vi "Lab Panel V4.91.vi"() -> ()   [LabVIEW 2013] (continued)
                }
              }
              frame #3 {
                # "LAB02-2"
                n2516 = case shown="True" w4752 {
                  tunnel: w4754 -> [_ w4767]
                  tunnel: w4751 -> [_ w4764]
                  tunnel: w4753 -> [_ w4763]
                  frame False {
                  }
                  frame True {
                    n2517 = local read "TEMP START LAB02-2"() -> (w4769:cluster{"TL":dbl, "TN":dbl})
                    n2518 = local read "FAIL LAB02-2"() -> (w4760:cluster{"LO":dbl, "HI":dbl})
                    n2519 = local read "TDMS LAB02-2"() -> (w4768:refnum<k34>)
                    n2520 = local read "SET LAB02-2"() -> (w4765:T5)
                    n2521 = local read "DISP LAB02-2"() -> (w4766:T4)
                    n2522 = local read "SIG LAB02-2"() -> (w4770:T2)
                    n2523 = local read "RESULT LAB02-2"() -> (w4757:bool)
                    n2524 = Bundle("FAIL LAB02-2"=w4760, "SIG LAB02-2"=w4770, "TEMP START LAB02-2"=w4769, "DISP LAB02-2"=w4766, "SET LAB02-2"=w4765, "TDMS LAB02-2"=w4768) -> (w4755:T35)  [unwired: 1 in]
                    n2525 = call "sub vi - cycle&temp fail v7.vi"("Amps Lo?"=w4767, "Input Cluster"=w4755, "SELECT"=w4764, "Amps Hi?"=w4763, "Result In"=w4757) -> ("(FAIL) out"=w4759:cluster{"FAIL LO":dbl, "FAIL HI":dbl}, "(DISP) out"=w4762:T4, "T-RISE"=w4756:cluster{"T-RISE (L)":dbl, "T-RISE (N)":dbl}, "Result Out"=w4758:bool, "file error"=w4761:errorcluster)  [unwired: 10 in]
                    n2526 = local write "TEMP RISE LAB02-2"(w4756) -> ()
                    n2527 = local write "FAIL LAB02-2"(w4759) -> ()
                    n2528 = local write "DISP LAB02-2"(w4762) -> ()
                    n2529 = local write "RESULT LAB02-2"(w4758) -> ()
                    n2530 = local write "data file error"(w4761) -> ()
                  }
                }
              }
              frame #4 {
                # "LAB03-1"
                n2531 = case shown="True" w4772 {
                  tunnel: w4774 -> [_ w4787]
                  tunnel: w4771 -> [_ w4784]
                  tunnel: w4773 -> [_ w4783]
                  frame False {
                  }
                  frame True {
                    n2532 = local read "TEMP START LAB03-1"() -> (w4789:cluster{"TL":dbl, "TN":dbl})
                    n2533 = local read "FAIL LAB03-1"() -> (w4780:cluster{"LO":dbl, "HI":dbl})
                    n2534 = local read "TDMS LAB03-1"() -> (w4788:refnum<k34>)
                    n2535 = local read "SET LAB03-1"() -> (w4785:T5)
                    n2536 = local read "DISP LAB03-1"() -> (w4786:T4)
                    n2537 = local read "SIG LAB03-1"() -> (w4790:T2)
                    n2538 = local read "RESULT LAB03-1"() -> (w4777:bool)
                    n2539 = Bundle("FAIL LAB03-1"=w4780, "SIG LAB03-1"=w4790, "TEMP START LAB03-1"=w4789, "DISP LAB03-1"=w4786, "SET LAB03-1"=w4785, "TDMS LAB03-1"=w4788) -> (w4775:T36)  [unwired: 1 in]
                    n2540 = call "sub vi - cycle&temp fail v7.vi"("Amps Lo?"=w4787, "Input Cluster"=w4775, "SELECT"=w4784, "Amps Hi?"=w4783, "Result In"=w4777) -> ("(FAIL) out"=w4779:cluster{"FAIL LO":dbl, "FAIL HI":dbl}, "(DISP) out"=w4782:T4, "T-RISE"=w4776:cluster{"T-RISE (L)":dbl, "T-RISE (N)":dbl}, "Result Out"=w4778:bool, "file error"=w4781:errorcluster)  [unwired: 10 in]
                    n2541 = local write "TEMP RISE LAB03-1"(w4776) -> ()
                    n2542 = local write "FAIL LAB03-1"(w4779) -> ()
                    n2543 = local write "DISP LAB03-1"(w4782) -> ()
                    n2544 = local write "RESULT LAB03-1"(w4778) -> ()
                    n2545 = local write "data file error"(w4781) -> ()
                  }
                }
              }
              frame #5 {
                # "LAB03-2"
                n2546 = case shown="True" w4792 {
                  tunnel: w4794 -> [_ w4807]
                  tunnel: w4791 -> [_ w4804]
                  tunnel: w4793 -> [_ w4803]
                  frame False {
                  }
                  frame True {
                    n2547 = local read "TEMP START LAB03-2"() -> (w4809:cluster{"TL":dbl, "TN":dbl})
                    n2548 = local read "FAIL LAB03-2"() -> (w4800:cluster{"LO":dbl, "HI":dbl})
                    n2549 = local read "TDMS LAB03-2"() -> (w4808:refnum<k34>)
                    n2550 = local read "SET LAB03-2"() -> (w4805:T5)
                    n2551 = local read "DISP LAB03-2"() -> (w4806:T4)
                    n2552 = local read "RESULT LAB03-2"() -> (w4797:bool)
                    n2553 = local read "SIG LAB03-2"() -> (w4810:T2)
                    n2554 = Bundle("FAIL LAB03-2"=w4800, "SIG LAB03-2"=w4810, "TEMP START LAB03-2"=w4809, "DISP LAB03-2"=w4806, "SET LAB03-2"=w4805, "TDMS LAB03-2"=w4808) -> (w4795:T37)  [unwired: 1 in]
                    n2555 = call "sub vi - cycle&temp fail v7.vi"("Amps Lo?"=w4807, "Input Cluster"=w4795, "SELECT"=w4804, "Amps Hi?"=w4803, "Result In"=w4797) -> ("(FAIL) out"=w4799:cluster{"FAIL LO":dbl, "FAIL HI":dbl}, "(DISP) out"=w4802:T4, "T-RISE"=w4796:cluster{"T-RISE (L)":dbl, "T-RISE (N)":dbl}, "Result Out"=w4798:bool, "file error"=w4801:errorcluster)  [unwired: 10 in]
                    n2556 = local write "FAIL LAB03-2"(w4799) -> ()
                    n2557 = local write "TEMP RISE LAB03-2"(w4796) -> ()
                    n2558 = local write "DISP LAB03-2"(w4802) -> ()
                    n2559 = local write "RESULT LAB03-2"(w4798) -> ()
                    n2560 = local write "data file error"(w4801) -> ()
                  }
                }
              }
              frame #6 {
                # "LAB04-1"
                n2561 = case shown="True" w4812 {
                  tunnel: w4814 -> [_ w4827]
                  tunnel: w4811 -> [_ w4824]
                  tunnel: w4813 -> [_ w4823]
                  frame False {
                  }
                  frame True {
                    n2562 = local read "TEMP START LAB04-1"() -> (w4829:cluster{"TL":dbl, "TN":dbl})
                    n2563 = local read "FAIL LAB04-1"() -> (w4820:cluster{"LO":dbl, "HI":dbl})
                    n2564 = local read "TDMS LAB04-1"() -> (w4828:refnum<k34>)
                    n2565 = local read "SET LAB04-1"() -> (w4825:T5)
                    n2566 = local read "DISP LAB04-1"() -> (w4826:T4)
                    n2567 = local read "SIG LAB04-1"() -> (w4830:T2)
                    n2568 = local read "RESULT LAB04-1"() -> (w4817:bool)
                    n2569 = Bundle("FAIL LAB04-1"=w4820, "SIG LAB04-1"=w4830, "TEMP START LAB04-1"=w4829, "DISP LAB04-1"=w4826, "SET LAB04-1"=w4825, "TDMS LAB04-1"=w4828) -> (w4815:T38)  [unwired: 1 in]
                    n2570 = call "sub vi - cycle&temp fail v7.vi"("Amps Lo?"=w4827, "Input Cluster"=w4815, "SELECT"=w4824, "Amps Hi?"=w4823, "Result In"=w4817) -> ("(FAIL) out"=w4819:cluster{"FAIL LO":dbl, "FAIL HI":dbl}, "(DISP) out"=w4822:T4, "T-RISE"=w4816:cluster{"T-RISE (L)":dbl, "T-RISE (N)":dbl}, "Result Out"=w4818:bool, "file error"=w4821:errorcluster)  [unwired: 10 in]
                    n2571 = local write "TEMP RISE LAB04-1"(w4816) -> ()
                    n2572 = local write "FAIL LAB04-1"(w4819) -> ()
                    n2573 = local write "DISP LAB04-1"(w4822) -> ()
                    n2574 = local write "RESULT LAB04-1"(w4818) -> ()
                    n2575 = local write "data file error"(w4821) -> ()
                  }
                }
              }
              frame #7 {
                # "LAB04-2"
                n2576 = case shown="True" w4832 {
                  tunnel: w4834 -> [_ w4847]
                  tunnel: w4831 -> [_ w4844]
                  tunnel: w4833 -> [_ w4843]
                  frame False {
                  }
                  frame True {
                    n2577 = local read "TEMP START LAB04-2"() -> (w4849:cluster{"TL":dbl, "TN":dbl})
                    n2578 = local read "FAIL LAB04-2"() -> (w4840:cluster{"LO":dbl, "HI":dbl})
                    n2579 = local read "TDMS LAB04-2"() -> (w4848:refnum<k34>)
                    n2580 = local read "SET LAB04-2"() -> (w4845:T5)
                    n2581 = local read "DISP LAB04-2"() -> (w4846:T4)
                    n2582 = local read "SIG LAB04-2"() -> (w4850:T2)
                    n2583 = local read "RESULT LAB04-2"() -> (w4837:bool)
                    n2584 = Bundle("FAIL LAB04-2"=w4840, "SIG LAB04-2"=w4850, "TEMP START LAB04-2"=w4849, "DISP LAB04-2"=w4846, "SET LAB04-2"=w4845, "TDMS LAB04-2"=w4848) -> (w4835:T39)  [unwired: 1 in]
                    n2585 = call "sub vi - cycle&temp fail v7.vi"("Amps Lo?"=w4847, "Input Cluster"=w4835, "SELECT"=w4844, "Amps Hi?"=w4843, "Result In"=w4837) -> ("(FAIL) out"=w4839:cluster{"FAIL LO":dbl, "FAIL HI":dbl}, "(DISP) out"=w4842:T4, "T-RISE"=w4836:cluster{"T-RISE (L)":dbl, "T-RISE (N)":dbl}, "Result Out"=w4838:bool, "file error"=w4841:errorcluster)  [unwired: 10 in]
                    n2586 = local write "TEMP RISE LAB04-2"(w4836) -> ()
                    n2587 = local write "FAIL LAB04-2"(w4839) -> ()
                    n2588 = local write "DISP LAB04-2"(w4842) -> ()
                    n2589 = local write "RESULT LAB04-2"(w4838) -> ()
                    n2590 = local write "data file error"(w4841) -> ()
                  }
                }
              }
              frame #8 {
                # "LAB05-1"
                n2591 = case shown="True" w4852 {
                  tunnel: w4854 -> [_ w4867]
                  tunnel: w4851 -> [_ w4864]
                  tunnel: w4853 -> [_ w4863]
                  frame False {
                  }
                  frame True {
                    n2592 = local read "TEMP START LAB05-1"() -> (w4869:cluster{"TL":dbl, "TN":dbl})
                    n2593 = local read "FAIL LAB05-1"() -> (w4860:cluster{"LO":dbl, "HI":dbl})
                    n2594 = local read "TDMS LAB05-1"() -> (w4868:refnum<k34>)
                    n2595 = local read "SET LAB05-1"() -> (w4865:T5)
                    n2596 = local read "DISP LAB05-1"() -> (w4866:T4)
                    n2597 = local read "SIG LAB05-1"() -> (w4870:T2)
                    n2598 = local read "RESULT LAB05-1"() -> (w4857:bool)
                    n2599 = Bundle("FAIL LAB05-1"=w4860, "SIG LAB05-1"=w4870, "TEMP START LAB05-1"=w4869, "DISP LAB05-1"=w4866, "SET LAB05-1"=w4865, "TDMS LAB05-1"=w4868) -> (w4855:T40)  [unwired: 1 in]
                    n2600 = call "sub vi - cycle&temp fail v7.vi"("Amps Lo?"=w4867, "Input Cluster"=w4855, "SELECT"=w4864, "Amps Hi?"=w4863, "Result In"=w4857) -> ("(FAIL) out"=w4859:cluster{"FAIL LO":dbl, "FAIL HI":dbl}, "(DISP) out"=w4862:T4, "T-RISE"=w4856:cluster{"T-RISE (L)":dbl, "T-RISE (N)":dbl}, "Result Out"=w4858:bool, "file error"=w4861:errorcluster)  [unwired: 10 in]
                    n2601 = local write "TEMP RISE LAB05-1"(w4856) -> ()
                    n2602 = local write "FAIL LAB05-1"(w4859) -> ()
                    n2603 = local write "DISP LAB05-1"(w4862) -> ()
                    n2604 = local write "RESULT LAB05-1"(w4858) -> ()
                    n2605 = local write "data file error"(w4861) -> ()
                  }
                }
              }
              frame #9 {
                # "LAB05-2"
                n2606 = case shown="True" w4872 {
                  tunnel: w4874 -> [_ w4887]
                  tunnel: w4871 -> [_ w4884]
                  tunnel: w4873 -> [_ w4883]
                  frame False {
                  }
                  frame True {
                    n2607 = local read "TEMP START LAB05-2"() -> (w4889:cluster{"TL":dbl, "TN":dbl})
                    n2608 = local read "FAIL LAB05-2"() -> (w4880:cluster{"LO":dbl, "HI":dbl})
                    n2609 = local read "TDMS LAB05-2"() -> (w4888:refnum<k34>)
                    n2610 = local read "SET LAB05-2"() -> (w4885:T5)
                    n2611 = local read "DISP LAB05-2"() -> (w4886:T4)
                    n2612 = local read "SIG LAB05-2"() -> (w4890:T2)
                    n2613 = local read "RESULT LAB05-2"() -> (w4877:bool)
                    n2614 = Bundle("FAIL LAB05-2"=w4880, "SIG LAB05-2"=w4890, "TEMP START LAB05-2"=w4889, "DISP LAB05-2"=w4886, "SET LAB05-2"=w4885, "TDMS LAB05-2"=w4888) -> (w4875:T41)  [unwired: 1 in]
                    n2615 = call "sub vi - cycle&temp fail v7.vi"("Amps Lo?"=w4887, "Input Cluster"=w4875, "SELECT"=w4884, "Amps Hi?"=w4883, "Result In"=w4877) -> ("(FAIL) out"=w4879:cluster{"FAIL LO":dbl, "FAIL HI":dbl}, "(DISP) out"=w4882:T4, "T-RISE"=w4876:cluster{"T-RISE (L)":dbl, "T-RISE (N)":dbl}, "Result Out"=w4878:bool, "file error"=w4881:errorcluster)  [unwired: 10 in]
                    n2616 = local write "TEMP RISE LAB05-2"(w4876) -> ()
                    n2617 = local write "FAIL LAB05-2"(w4879) -> ()
                    n2618 = local write "DISP LAB05-2"(w4882) -> ()
                    n2619 = local write "RESULT LAB05-2"(w4878) -> ()
                    n2620 = local write "data file error"(w4881) -> ()
                  }
                }
              }
            }
          }
          frame #15 {
            # "run calibration routine"
            n2621 = local read "SET (cal)"() -> (w4891:bool)
            n2622 = case shown="True" w4891 {
              frame False {
              }
              frame True {
                n2623 = stacked-sequence {
                  seq-local: [w4892 _ _] -> [_ w4894 _]
                  frame #0 {
                    n2624 = call "CALIBRATION PASSWORD"() -> ("PASSWORD"=w4892:string)  [unwired: 17 in, 2 out]
                  }
                  frame #1 {
                    n2625 = Equal?(x=w4894, y="7777") -> (x = y?=w4893:bool)
                    n2626 = case shown="True" w4893 {
                      frame False {
                      }
                      frame True {
                        n2627 = stacked-sequence {
                          frame #0 {
                            n2628 = local read "Temp Test Cal"() -> (w4896:dbl)
                            n2629 = call "sub vi - calibration v1.vi"("Temp Test Cal"=w4896) -> ()  [unwired: 11 in]
                          }
                          frame #1 {
                            n2630 = call "sub vi - get calibration values v1.vi"() -> ("TEMP REF CAL"=w4897:dbl, "LAB01 (CAL)"=w4902:T14, "LAB02 (CAL)"=w4901:T15, "LAB03 (CAL)"=w4900:T14, "LAB04 (CAL)"=w4899:T14, "calibration file error out"=w4903:errorcluster, "LAB05 (CAL)"=w4898:T14)  [unwired: 9 in]
                            n2631 = local write "TEMP REF cal"(w4897) -> ()
                            n2632 = local write "cal file error out"(w4903) -> ()
                            n2633 = local write "CAL LAB04"(w4899) -> ()
                            n2634 = local write "CAL LAB05"(w4898) -> ()
                            n2635 = local write "CAL LAB01"(w4902) -> ()
                            n2636 = local write "CAL LAB02"(w4901) -> ()
                            n2637 = local write "CAL LAB03"(w4900) -> ()
                          }
                        }
                      }
                    }
                  }
                  frame #2 {
                    n2638 = local write "SET (cal)"(FALSE) -> ()
                  }
                }
              }
            }
          }
          frame #16 {
            # "save certain settings to file"
            n2639 = String To Path(string="c:\\crabtree\\Set Up\\") -> (path=w4906:path)
            n2640 = Build Path(base path=w4906, name or relative path="settings.bin") -> (appended path=w4908:path)
            n2641 = Build Path(base path=w4906, name or relative path="mail.bin") -> (appended path=w4905:path)
            n2642 = Create Folder(path (use dialog)=w4906) -> (error out=w4911:errorcluster)  [unwired: 2 in, 2 out]
            n2643 = call <vilib>:"Clear Errors.vi"("error in (no error)"=w4911) -> ()  [unwired: 6 in, 1 out]
            n2644 = stacked-sequence {
              seq-local: [w4923 _] -> [_ w4936]
              tunnel: w4908 -> [_ w4937]
              tunnel: w4905 -> [_ w4935]
              frame #0 {
                n2645 = local read "C drive data root dir"() -> (w4922:path)
                n2646 = local read "Select COM port"() -> (w4919:refnum<visa-resource-name>)
                n2647 = local read "Network Directory"() -> (w4928:path)
                n2648 = local read "SET LAB05-2"() -> (w4927:T5)
                n2649 = local read "SET LAB05-1"() -> (w4926:T5)
                n2650 = local read "SET LAB04-2"() -> (w4925:T5)
                n2651 = local read "SET LAB03-2"() -> (w4929:T5)
                n2652 = local read "SET LAB04-1"() -> (w4924:T5)
                n2653 = local read "SET LAB03-1"() -> (w4930:T5)
                n2654 = local read "SET LAB02-2"() -> (w4931:T5)
                n2655 = local read "SET LAB02-1"() -> (w4932:T5)
                n2656 = local read "Temp Delay Lps"() -> (w4918:dbl)
                n2657 = local read "Amps Fail level"() -> (w4914:dbl)
                n2658 = local read "SET LAB01-2"() -> (w4933:T5)
                n2659 = local read "Temp Test Cal"() -> (w4915:dbl)
                n2660 = local read "SET LAB01-1"() -> (w4934:T5)
                n2661 = local read "Mail Test File To:"() -> (w4913:string)
                n2662 = local read "Temp Value"() -> (w4917:dbl)
                n2663 = local read "Fail Loops"() -> (w4916:dbl)
                n2664 = local read "Mail Test Fail"() -> (w4912:bool)
                n2665 = local read "RATE (Hz)"() -> (w4921:dbl)
                n2666 = local read "SAMPLES"() -> (w4920:dbl)
                n2667 = Bundle("SET LAB01-1"=w4934, "SET LAB01-2"=w4933, "SET LAB02-1"=w4932, "SET LAB02-2"=w4931, "SET LAB03-1"=w4930, "SET LAB03-2"=w4929, "SET LAB04-1"=w4924, "SET LAB04-2"=w4925, "SET LAB05-1"=w4926, "SET LAB05-2"=w4927, "Network Directory"=w4928, "C drive data root dir"=w4922, "RATE (Hz)"=w4921, "SAMPLES"=w4920, "Select COM port"=w4919, "Temp Delay Lps"=w4918, "Temp Value"=w4917, "Fail Loops"=w4916, "Temp Test Cal"=w4915, "Amps Fail level"=w4914, "Mail Test File To:"=w4913, "Mail Test Fail"=w4912) -> (w4923:T22)  [unwired: 1 in]
              }
              frame #1 {
                n2668 = event shown="[1] \"SET LAB01-1\", \"SET LAB01-2\", \"SET LAB02-1\", \"SET LAB02-2\", \"SET LAB03-1\", \"SET LAB03-2\", \"SET LAB04-1\", \"SET LAB04-2\", \"SET LAB05-1\", \"SET LAB05-2\", \"Network Directory\", \"C drive data root dir\", \"RATE (Hz)\", \"SAMPLES\", \"Select COM port\", \"Temp Delay Lps\", \"Temp Value\", \"Fail Loops\", \"Temp Test Cal\", \"Amps Fail level\", \"Mail Test File To:\", \"Mail Test Fail\": Value Change" {
                  selector: _ -> [_ _ _]
                  dyn-events: _ -> [_ _ _]
                  timeout: 10.0 -> [_ _ _]
                  tunnel: w4937 -> [_ w4939 _]
                  tunnel: w4936 -> [_ w4940 _]
                  tunnel: w4935 -> [_ _ w4951]
                  event Timeout {
                    n2669 = event-data() -> ()  [unwired: 1 in, 3 out]
                  }
                  event "SET LAB01-1", "SET LAB01-2", "SET LAB02-1", "SET LAB02-2", "SET LAB03-1", "SET LAB03-2", "SET LAB04-1", "SET LAB04-2", "SET LAB05-1", "SET LAB05-2", "Network Directory", "C drive data root dir", "RATE (Hz)", "SAMPLES", "Select COM port", "Temp Delay Lps", "Temp Value", "Fail Loops", "Temp Test Cal", "Amps Fail level", "Mail Test File To:", "Mail Test Fail": Value Change {
                    n2670 = event-data() -> ()  [unwired: 1 in, 6 out]
                    n2671 = Open/Create/Replace File(file path (use dialog)=w4939, operation (0:open)=T21."replace or create") -> (refnum out=w4945:refnum<file>, error out=w4944:errorcluster)  [unwired: 4 in, 1 out]
                    n2672 = Write to Binary File(file (use dialog)=w4945, data=w4940, error in=w4944) -> (refnum out=w4943:refnum<file>, error out=w4942:errorcluster)  [unwired: 3 in, 1 out]
                    n2673 = Close File(refnum=w4943, error in=w4942) -> (error out=w4941:errorcluster)  [unwired: 1 out]
                    n2674 = local write "data file error"(w4941) -> ()
                  }
                  event "MAIL SETTINGS.OUT SERVER ADDRESS", "MAIL SETTINGS.FROM ACCOUNT", "MAIL SETTINGS.USER NAME", "MAIL SETTINGS.PASSWORD", "Auto Mail Send", "TO (string):": Value Change {
                    n2675 = event-data() -> ()  [unwired: 1 in, 6 out]
                    n2676 = local read "MAIL SETTINGS"() -> (w4950:T7)
                    n2677 = local read "Auto Mail Send"() -> (w4948:bool)
                    n2678 = local read "TO (string):"() -> (w4947:string)
                    n2679 = Open/Create/Replace File(file path (use dialog)=w4951, operation (0:open)=T21."replace or create") -> (refnum out=w4956:refnum<file>, error out=w4955:errorcluster)  [unwired: 4 in, 1 out]
                    n2680 = Bundle("MAIL SETTINGS"=w4950, "Auto Mail Send"=w4948, "TO (string):"=w4947) -> (w4949:T42)  [unwired: 1 in]
                    n2681 = Write to Binary File(file (use dialog)=w4956, data=w4949, error in=w4955) -> (refnum out=w4954:refnum<file>, error out=w4953:errorcluster)  [unwired: 3 in, 1 out]
                    n2682 = Close File(refnum=w4954, error in=w4953) -> (error out=w4952:errorcluster)  [unwired: 1 out]
                    n2683 = local write "data file error"(w4952) -> ()
                  }
                }
              }
            }
          }
          frame #17 {
            # "mail control"
            n2684 = local read "MAIL SETTINGS"() -> (w4973:T7)
            n2685 = local read "Auto Mail Send"() -> (w4959:bool)
            n2686 = Unbundle(w4973) -> ("OUT SERVER ADDRESS"=w4972:string, "FROM ACCOUNT"=w4971:string, "TEST MAIL"=w4970:bool)  [unwired: 4 out]
            n2687 = stacked-sequence {
              tunnel: "TO (string):" -> [_ w5012]
              tunnel: w4973 -> [w4978 w5011]
              tunnel: w4972 -> [w4977 w5010]
              tunnel: w4971 -> [w4976 w5009]
              tunnel: w4970 -> [w4975 _]
              tunnel: w4959 -> [_ w5008]
              tunnel: w4969 -> [_ w5007]
              tunnel: w4968 -> [_ w5006]
              tunnel: w4967 -> [_ w5005]
              tunnel: w4966 -> [_ w5004]
              tunnel: w4965 -> [_ w5003]
              tunnel: w4964 -> [_ w5002]
              tunnel: w4963 -> [_ w5001]
              tunnel: w4962 -> [_ w5000]
              tunnel: w4961 -> [_ w4999]
              tunnel: w4960 -> [_ w4998]
              tunnel: "TO (string):" -> [w4974 _]
              frame #0 {
                # "mail test"
                n2688 = case shown="True" w4975 {
                  tunnel: w4978 -> [_ w4982]
                  tunnel: w4974 -> [_ w4981]
                  tunnel: w4977 -> [_ w4980]
                  tunnel: w4976 -> [_ w4979]
                  frame False {
                  }
                  frame True {
                    n2689 = stacked-sequence {
                      seq-local: [_ _ w4992 _] -> [_ _ _ w4993]
                      tunnel: w4982 -> [w4985 _ _ w4997]
                      tunnel: w4981 -> [_ _ w4990 _]
                      tunnel: w4980 -> [_ _ w4988 _]
                      tunnel: w4979 -> [_ _ w4989 _]
                      frame #0 {
                        n2690 = Bundle(cluster=w4985, "TEST MAIL STATUS"="TEST START") -> (w4983:T7)  [unwired: 6 in]
                        n2691 = local write "MAIL SETTINGS"(w4983) -> ()
                      }
                      frame #1 {
                        n2692 = Wait (ms)(milliseconds to wait=500) -> ()  [unwired: 1 out]
                      }
                      frame #2 {
                        n2693 = call "sub vi - send mail v5.vi"("TO:"=w4990, "subject"="MAIL TEST FROM LAB PANEL", "from"=w4989, "out going server"=w4988, "message"="TEST MESSAGE") -> ("error out"=w4992:errorcluster)  [unwired: 10 in]
                      }
                      frame #3 {
                        n2694 = Bundle(cluster=w4997, "TEST MAIL"=FALSE, "TEST MAIL STATUS"="TEST END", "mail error"=w4993) -> (w4995:T7)  [unwired: 4 in]
                        n2695 = local write "MAIL SETTINGS"(w4995) -> ()
                      }
                    }
                  }
                }
              }
              frame #1 {
                # "mail report"
                n2696 = stacked-sequence {
                  seq-local: [_ w5055 _ _] -> [_ _ _ w5245]
                  seq-local: [_ _ w5158 _] -> [_ _ _ w5235]
                  seq-local: [w5022 _ _ _] -> [_ w5072 _ _]
                  seq-local: [w5021 _ _ _] -> [_ w5071 _ _]
                  seq-local: [w5019 _ _ _] -> [_ w5069 _ _]
                  seq-local: [w5020 _ _ _] -> [_ w5070 _ _]
                  seq-local: [w5018 _ _ _] -> [_ w5068 _ _]
                  seq-local: [w5017 _ _ _] -> [_ w5063 _ _]
                  seq-local: [w5016 _ _ _] -> [_ w5064 _ _]
                  seq-local: [w5015 _ _ _] -> [_ w5065 _ _]
                  seq-local: [w5014 _ _ _] -> [_ w5066 _ _]
                  seq-local: [w5013 _ _ _] -> [_ w5067 _ _]
                  tunnel: w5012 -> [_ _ _ w5246]
                  tunnel: w5011 -> [_ _ _ w5229]
                  tunnel: w5010 -> [_ _ _ w5243]
                  tunnel: w5009 -> [_ _ _ w5242]
                  tunnel: w5008 -> [w5053 _ _ w5237]
                  tunnel: w5007 -> [_ _ w5188 _]
                  tunnel: w5006 -> [_ _ w5185 _]
                  tunnel: w5005 -> [_ _ w5184 _]
                  tunnel: w5004 -> [_ _ w5183 _]
                  tunnel: w5003 -> [_ _ w5182 _]
                  tunnel: w5002 -> [_ _ w5181 _]
                  tunnel: w5001 -> [_ _ w5180 _]
                  tunnel: w5000 -> [_ _ w5179 _]
                  tunnel: w4999 -> [_ _ w5178 _]
                  tunnel: w4998 -> [_ _ w5177 _]
                  frame #0 {
                    n2697 = case shown="False" w5053 {
                      frame False {
                        n2698 = local write "mail control"("") -> ()
                      }
                      frame True {
                      }
                    }
                    n2699 = local read "SET LAB01-1"() -> (w5052:T5)
                    n2700 = local read "SET LAB01-2"() -> (w5051:T5)
                    n2701 = local read "SET LAB02-1"() -> (w5050:T5)
                    n2702 = local read "SET LAB02-2"() -> (w5049:T5)
                    n2703 = local read "SET LAB03-1"() -> (w5048:T5)
                    n2704 = local read "SET LAB04-1"() -> (w5046:T5)
                    n2705 = local read "SET LAB05-1"() -> (w5044:T5)
                    n2706 = local read "SET LAB03-2"() -> (w5047:T5)
                    n2707 = local read "SET LAB04-2"() -> (w5045:T5)
                    n2708 = local read "SET LAB05-2"() -> (w5043:T5)
                    n2709 = Unbundle(w5048) -> ("DESCRIPTION"=w5028:string)  [unwired: 4 out]
                    n2710 = Unbundle(w5047) -> ("DESCRIPTION"=w5027:string)  [unwired: 4 out]
                    n2711 = Unbundle(w5046) -> ("DESCRIPTION"=w5026:string)  [unwired: 4 out]
                    n2712 = Unbundle(w5043) -> ("DESCRIPTION"=w5023:string)  [unwired: 4 out]
                    n2713 = Unbundle(w5049) -> ("DESCRIPTION"=w5029:string)  [unwired: 4 out]
                    n2714 = Unbundle(w5045) -> ("DESCRIPTION"=w5025:string)  [unwired: 4 out]
                    n2715 = Unbundle(w5052) -> ("DESCRIPTION"=w5041:string)  [unwired: 4 out]
                    n2716 = Unbundle(w5050) -> ("DESCRIPTION"=w5030:string)  [unwired: 4 out]
                    n2717 = Unbundle(w5044) -> ("DESCRIPTION"=w5024:string)  [unwired: 4 out]
                    n2718 = Unbundle(w5051) -> ("DESCRIPTION"=w5031:string)  [unwired: 4 out]
                    n2719 = Concatenate Strings("[LAB05-2/", w5023) -> (w5013:string)
                    n2720 = Concatenate Strings("[LAB05-1/", w5024) -> (w5014:string)
                    n2721 = Concatenate Strings("[LAB04-2/", w5025) -> (w5015:string)
                    n2722 = Concatenate Strings("[LAB03-2/", w5027) -> (w5017:string)
                    n2723 = Concatenate Strings("[LAB04-1/", w5026) -> (w5016:string)
                    n2724 = Concatenate Strings("[LAB03-1/", w5028) -> (w5018:string)
                    n2725 = Concatenate Strings("[LAB01-2/", w5031) -> (w5021:string)
                    n2726 = Concatenate Strings("[LAB02-2/", w5029) -> (w5019:string)
                    n2727 = Concatenate Strings("[LAB01-1/", w5041) -> (w5022:string)
                    n2728 = Concatenate Strings("[LAB02-1/", w5030) -> (w5020:string)
                  }
                  frame #1 {
                    w5076 = "/"
                    w5077 = 2.0
                    n2729 = local read "DISP LAB01-2"() -> (w5156:T4)
                    n2730 = local read "DISP LAB01-1"() -> (w5157:T4)
                    n2731 = local read "DISP LAB02-1"() -> (w5155:T4)
                    n2732 = local read "DISP LAB03-2"() -> (w5152:T4)
                    n2733 = local read "DISP LAB02-2"() -> (w5154:T4)
                    n2734 = local read "DISP LAB03-1"() -> (w5153:T4)
                    n2735 = local read "DISP LAB04-2"() -> (w5150:T4)
                    n2736 = local read "DISP LAB04-1"() -> (w5151:T4)
                    n2737 = local read "DISP LAB05-1"() -> (w5149:T4)
                    n2738 = local read "DISP LAB05-2"() -> (w5148:T4)
                    n2739 = Unbundle(w5156) -> ("CYCLE"=w5140:dbl, "MINS"=w5139:dbl, "STATUS"=w5136:string)
                    n2740 = Unbundle(w5157) -> ("CYCLE"=w5145:dbl, "MINS"=w5144:dbl, "STATUS"=w5141:string)
                    n2741 = Unbundle(w5155) -> ("CYCLE"=w5133:dbl, "MINS"=w5132:dbl, "STATUS"=w5131:string)
                    n2742 = Unbundle(w5152) -> ("CYCLE"=w5120:dbl, "MINS"=w5119:dbl, "STATUS"=w5116:string)
                    n2743 = Unbundle(w5153) -> ("CYCLE"=w5125:dbl, "MINS"=w5124:dbl, "STATUS"=w5121:string)
                    n2744 = Unbundle(w5154) -> ("CYCLE"=w5130:dbl, "MINS"=w5129:dbl, "STATUS"=w5126:string)
                    n2745 = Unbundle(w5151) -> ("CYCLE"=w5115:dbl, "MINS"=w5114:dbl, "STATUS"=w5111:string)
                    n2746 = Unbundle(w5150) -> ("CYCLE"=w5110:dbl, "MINS"=w5109:dbl, "STATUS"=w5106:string)
                    n2747 = Unbundle(w5149) -> ("CYCLE"=w5105:dbl, "MINS"=w5104:dbl, "STATUS"=w5101:string)
                    n2748 = Unbundle(w5148) -> ("CYCLE"=w5147:dbl, "MINS"=w5146:dbl, "STATUS"=w5098:string)
                    n2749 = Number To Decimal String(number=w5133) -> (decimal integer string=w5135:string)  [unwired: 1 in]
                    n2750 = Number To Decimal String(number=w5130) -> (decimal integer string=w5128:string)  [unwired: 1 in]
                    n2751 = Number To Decimal String(number=w5125) -> (decimal integer string=w5123:string)  [unwired: 1 in]
                    n2752 = Number To Decimal String(number=w5140) -> (decimal integer string=w5138:string)  [unwired: 1 in]
                    n2753 = Number To Decimal String(number=w5120) -> (decimal integer string=w5118:string)  [unwired: 1 in]
                    n2754 = Number To Decimal String(number=w5145) -> (decimal integer string=w5143:string)  [unwired: 1 in]
                    n2755 = Number To Decimal String(number=w5147) -> (decimal integer string=w5100:string)  [unwired: 1 in]
                    n2756 = Number To Decimal String(number=w5115) -> (decimal integer string=w5113:string)  [unwired: 1 in]
                    n2757 = Number To Decimal String(number=w5110) -> (decimal integer string=w5108:string)  [unwired: 1 in]
                    n2758 = Number To Decimal String(number=w5105) -> (decimal integer string=w5103:string)  [unwired: 1 in]
                    n2759 = Number To Fractional String(number=w5132, precision (6)=w5077) -> (F-format string=w5134:string)  [unwired: 2 in]
                    n2760 = Number To Fractional String(number=w5119, precision (6)=w5077) -> (F-format string=w5117:string)  [unwired: 2 in]
                    n2761 = Number To Fractional String(number=w5129, precision (6)=w5077) -> (F-format string=w5127:string)  [unwired: 2 in]
                    n2762 = Number To Fractional String(number=w5124, precision (6)=w5077) -> (F-format string=w5122:string)  [unwired: 2 in]
                    n2763 = Number To Fractional String(number=w5109, precision (6)=w5077) -> (F-format string=w5107:string)  [unwired: 2 in]
                    n2764 = Number To Fractional String(number=w5114, precision (6)=w5077) -> (F-format string=w5112:string)  [unwired: 2 in]
                    n2765 = Number To Fractional String(number=w5139, precision (6)=w5077) -> (F-format string=w5137:string)  [unwired: 2 in]
                    n2766 = Number To Fractional String(number=w5104, precision (6)=w5077) -> (F-format string=w5102:string)  [unwired: 2 in]
                    n2767 = Number To Fractional String(number=w5144, precision (6)=w5077) -> (F-format string=w5142:string)  [unwired: 2 in]
                    n2768 = Number To Fractional String(number=w5146, precision (6)=w5077) -> (F-format string=w5099:string)  [unwired: 2 in]
                    n2769 = Concatenate Strings(w5076, w5118, w5076, w5117, w5076, w5116) -> (w5092:string)
                    n2770 = Concatenate Strings(w5076, w5113, w5076, w5112, w5076, w5111) -> (w5091:string)
                    n2771 = Concatenate Strings(w5076, w5108, w5076, w5107, w5076, w5106) -> (w5090:string)
                    n2772 = Concatenate Strings(w5076, w5103, w5076, w5102, w5076, w5101) -> (w5089:string)
                    n2773 = Concatenate Strings(w5076, w5100, w5076, w5099, w5076, w5098) -> (w5088:string)
                    n2774 = Concatenate Strings(w5076, w5143, w5076, w5142, w5076, w5141) -> (w5097:string)
                    n2775 = Concatenate Strings(w5076, w5123, w5076, w5122, w5076, w5121) -> (w5093:string)
                    n2776 = Concatenate Strings(w5076, w5138, w5076, w5137, w5076, w5136) -> (w5096:string)
                    n2777 = Concatenate Strings(w5076, w5135, w5076, w5134, w5076, w5131) -> (w5095:string)
                    n2778 = Concatenate Strings(w5076, w5128, w5076, w5127, w5076, w5126) -> (w5094:string)
                    n2779 = Concatenate Strings("]", "\r") -> (w5073:string)
                    n2780 = Concatenate Strings(w5068, w5093, w5073) -> (w5083:string)
                    n2781 = Concatenate Strings(w5070, w5095, w5073) -> (w5085:string)
                    n2782 = Concatenate Strings(w5069, w5094, w5073) -> (w5084:string)
                    n2783 = Concatenate Strings(w5065, w5090, w5073) -> (w5080:string)
                    n2784 = Concatenate Strings(w5066, w5089, w5073) -> (w5081:string)
                    n2785 = Concatenate Strings(w5064, w5091, w5073) -> (w5079:string)
                    n2786 = Concatenate Strings(w5063, w5092, w5073) -> (w5078:string)
                    n2787 = Concatenate Strings(w5067, w5088, w5073) -> (w5082:string)
                    n2788 = Concatenate Strings(w5071, w5096, w5073) -> (w5086:string)
                    n2789 = Concatenate Strings(w5072, w5097, w5073) -> (w5087:string)
                    n2790 = Concatenate Strings(w5087, w5086, w5085, w5084, w5083, w5078, w5079, w5080, w5081, w5082) -> (w5056:string)
                    n2791 = Concatenate Strings("[PANEL/", "DESC/", "CYCLES/", "MINS/", "STATUS]", "\r", w5056) -> (w5055:string)
                    "MAIL REPORT" <- w5055
                    n2792 = global write "Global display 3.vi" "log all"(w5055) -> ()
                  }
                  frame #2 {
                    w5186 = "END"
                    n2793 = local read "mail control"() -> (w5187:string)
                    n2794 = case shown="False" w5182 {
                      tunnel: w5187 -> [w5211 _]
                      tunnel: w5186 -> [w5210 _]
                      tunnel: [w5209 FALSE] -> w5172
                      frame False {
                        n2795 = Equal?(x=w5211, y=w5210) -> (x = y?=w5209:bool)
                      }
                      frame True {
                      }
                    }
                    n2796 = case shown="False" w5188 {
                      tunnel: w5187 -> [w5227 _]
                      tunnel: w5186 -> [w5226 _]
                      tunnel: [w5225 FALSE] -> w5176
                      frame False {
                        n2797 = Equal?(x=w5227, y=w5226) -> (x = y?=w5225:bool)
                      }
                      frame True {
                      }
                    }
                    n2798 = case shown="False" w5185 {
                      tunnel: w5187 -> [w5223 _]
                      tunnel: w5186 -> [w5222 _]
                      tunnel: [w5221 FALSE] -> w5175
                      frame False {
                        n2799 = Equal?(x=w5223, y=w5222) -> (x = y?=w5221:bool)
                      }
                      frame True {
                      }
                    }
                    n2800 = case shown="False" w5183 {
                      tunnel: w5187 -> [w5215 _]
                      tunnel: w5186 -> [w5214 _]
                      tunnel: [w5213 FALSE] -> w5173
                      frame False {
                        n2801 = Equal?(x=w5215, y=w5214) -> (x = y?=w5213:bool)
                      }
                      frame True {
                      }
                    }
                    n2802 = case shown="False" w5184 {
                      tunnel: w5187 -> [w5219 _]
                      tunnel: w5186 -> [w5218 _]
                      tunnel: [w5217 FALSE] -> w5174
                      frame False {
                        n2803 = Equal?(x=w5219, y=w5218) -> (x = y?=w5217:bool)
                      }
                      frame True {
                      }
                    }
                    n2804 = Or(x=w5174, y=w5173) -> (x .or. y?=w5165:bool)
                    n2805 = Or(x=w5176, y=w5175) -> (x .or. y?=w5166:bool)
                    n2806 = Or(x=w5166, y=w5165) -> (x .or. y?=w5161:bool)
                    n2807 = case shown="False" w5178 {
                      tunnel: w5187 -> [w5195 _]
                      tunnel: w5186 -> [w5194 _]
                      tunnel: [w5193 FALSE] -> w5167
                      frame False {
                        n2808 = Equal?(x=w5195, y=w5194) -> (x = y?=w5193:bool)
                      }
                      frame True {
                      }
                    }
                    n2809 = case shown="False" w5177 {
                      tunnel: w5187 -> [w5191 _]
                      tunnel: w5186 -> [w5190 _]
                      tunnel: [w5189 FALSE] -> w5171
                      frame False {
                        n2810 = Equal?(x=w5191, y=w5190) -> (x = y?=w5189:bool)
                      }
                      frame True {
                      }
                    }
                    n2811 = case shown="False" w5179 {
                      tunnel: w5187 -> [w5199 _]
                      tunnel: w5186 -> [w5198 _]
                      tunnel: [w5197 FALSE] -> w5168
                      frame False {
                        n2812 = Equal?(x=w5199, y=w5198) -> (x = y?=w5197:bool)
                      }
                      frame True {
                      }
                    }
                    n2813 = case shown="False" w5181 {
                      tunnel: w5187 -> [w5207 _]
                      tunnel: w5186 -> [w5206 _]
                      tunnel: [w5205 FALSE] -> w5170
                      frame False {
                        n2814 = Equal?(x=w5207, y=w5206) -> (x = y?=w5205:bool)
                      }
                      frame True {
                      }
                    }
                    n2815 = case shown="False" w5180 {
                      tunnel: w5187 -> [w5203 _]
                      tunnel: w5186 -> [w5202 _]
                      tunnel: [w5201 FALSE] -> w5169
                      frame False {
                        n2816 = Equal?(x=w5203, y=w5202) -> (x = y?=w5201:bool)
                      }
                      frame True {
                      }
                    }
                    n2817 = Or(x=w5170, y=w5169) -> (x .or. y?=w5164:bool)
                    n2818 = Or(x=w5168, y=w5167) -> (x .or. y?=w5163:bool)
                    n2819 = Or(x=w5171, y=w5172) -> (x .or. y?=w5159:bool)
                    n2820 = Or(x=w5164, y=w5163) -> (x .or. y?=w5162:bool)
                    n2821 = Or(x=w5161, y=w5162) -> (x .or. y?=w5160:bool)
                    n2822 = Or(x=w5160, y=w5159) -> (x .or. y?=w5158:bool)
                  }
                  frame #3 {
                    n2823 = local read "on loops"() -> (w5241:dbl)
                    n2824 = local read "jig cycle"() -> (w5238:dbl)
                    n2825 = local read "Send Mail Now"() -> (w5232:bool)
                    n2826 = Add(x=w5241, y=3.0) -> (x+y=w5239:dbl)
                    n2827 = Equal?(x=w5238, y=w5239) -> (x = y?=w5233:bool)
                    n2828 = And(x=w5233, y=w5232) -> (x .and. y?=w5231:bool)
                    n2829 = And(x=w5237, y=w5233) -> (x .and. y?=w5236:bool)
                    n2830 = And(x=w5236, y=w5235) -> (x .and. y?=w5234:bool)
                    n2831 = Or(x=w5234, y=w5231) -> (x .or. y?=w5230:bool)
                    n2832 = case shown="True" w5230 {
                      tunnel: w5246 -> [_ w5252]
                      tunnel: w5245 -> [_ w5251]
                      tunnel: "Lab Panel Test Status" -> [_ w5250]
                      tunnel: w5243 -> [_ w5249]
                      tunnel: w5242 -> [_ w5248]
                      tunnel: w5229 -> [_ w5247]
                      frame False {
                      }
                      frame True {
                        n2833 = stacked-sequence {
                          tunnel: w5252 -> [w5260 _]
                          tunnel: w5251 -> [w5259 _]
                          tunnel: w5250 -> [w5258 _]
                          tunnel: w5249 -> [w5257 _]
                          tunnel: w5248 -> [w5256 _]
                          tunnel: w5247 -> [w5255 _]
                          frame #0 {
                            n2834 = call "sub vi - send mail v5.vi"("TO:"=w5260, "subject"=w5258, "from"=w5256, "out going server"=w5257, "message"=w5259) -> ("error out"=w5254:errorcluster)  [unwired: 10 in]
                            n2835 = Bundle(cluster=w5255, "mail error"=w5254) -> (w5253:T7)  [unwired: 6 in]
                            n2836 = local write "MAIL SETTINGS"(w5253) -> ()
                          }
                          frame #1 {
                            n2837 = local write "mail control"("") -> ()
                            n2838 = local write "Send Mail Now"(FALSE) -> ()
                          }
                        }
                      }
                    }
                  }
                }
              }
            }
          }
          frame #18 {
            # "save jig cycle values once all run switches are off"
            n2839 = stacked-sequence {
              tunnel: w5272 -> [_ w5301]
              tunnel: w5271 -> [_ w5300]
              tunnel: w5270 -> [_ w5299]
              tunnel: w5269 -> [_ w5298]
              tunnel: w5268 -> [_ w5297]
              tunnel: w5267 -> [_ w5296]
              tunnel: w5266 -> [_ w5295]
              tunnel: w5265 -> [_ w5294]
              tunnel: w5264 -> [_ w5293]
              tunnel: w5263 -> [_ w5292]
              frame #0 {
              }
              frame #1 {
                n2840 = Not(x=w5292) -> (.not. x?=w5275:bool)
                n2841 = Not(x=w5300) -> (.not. x?=w5290:bool)
                n2842 = Not(x=w5297) -> (.not. x?=w5285:bool)
                n2843 = Not(x=w5295) -> (.not. x?=w5281:bool)
                n2844 = Not(x=w5293) -> (.not. x?=w5277:bool)
                n2845 = Not(x=w5301) -> (.not. x?=w5291:bool)
                n2846 = Not(x=w5299) -> (.not. x?=w5289:bool)
                n2847 = Not(x=w5296) -> (.not. x?=w5283:bool)
                n2848 = Not(x=w5298) -> (.not. x?=w5287:bool)
                n2849 = Not(x=w5294) -> (.not. x?=w5279:bool)
                n2850 = local read "Save JC"() -> (w5303:bool)
                n2851 = And(x=w5291, y=w5290) -> (x .and. y?=w5288:bool)
                n2852 = And(x=w5288, y=w5289) -> (x .and. y?=w5286:bool)
                n2853 = And(x=w5286, y=w5287) -> (x .and. y?=w5284:bool)
                n2854 = And(x=w5284, y=w5285) -> (x .and. y?=w5282:bool)
                n2855 = And(x=w5282, y=w5283) -> (x .and. y?=w5280:bool)
                n2856 = And(x=w5280, y=w5281) -> (x .and. y?=w5278:bool)
                n2857 = And(x=w5278, y=w5279) -> (x .and. y?=w5276:bool)
                n2858 = And(x=w5276, y=w5277) -> (x .and. y?=w5274:bool)
                n2859 = And(x=w5274, y=w5275) -> (x .and. y?=w5273:bool)
                n2860 = And(x=w5273, y=w5303) -> (x .and. y?=w5302:bool)
                n2861 = case shown="True" w5302 {
                  tunnel: w5273 -> [w5304 _]
                  frame False {
                    n2862 = case shown="False" w5304 {
                      frame False {
                        n2863 = local write "Save JC"(TRUE) -> ()
                      }
                      frame True {
                      }
                    }
                  }
                  frame True {
                    n2864 = stacked-sequence {
                      frame #0 {
                        n2865 = String To Path(string="c:\\crabtree\\Jig Cycles\\") -> (path=w5316:path)
                        n2866 = Build Path(base path=w5316, name or relative path="jigcycles.bin") -> (appended path=w5314:path)
                        n2867 = Create Folder(path (use dialog)=w5316) -> (error out=w5318:errorcluster)  [unwired: 2 in, 2 out]
                        n2868 = local read "JIG RELAY CYCLES"() -> (w5308:T8)
                        n2869 = call <vilib>:"Clear Errors.vi"("error in (no error)"=w5318) -> ()  [unwired: 6 in, 1 out]
                        n2870 = local write "Save JC"(FALSE) -> ()
                        n2871 = Open/Create/Replace File(file path (use dialog)=w5314, operation (0:open)=T21."replace or create") -> (refnum out=w5312:refnum<file>, error out=w5313:errorcluster)  [unwired: 4 in, 1 out]
                        n2872 = Write to Binary File(file (use dialog)=w5312, data=w5308, error in=w5313) -> (refnum out=w5311:refnum<file>, error out=w5310:errorcluster)  [unwired: 3 in, 1 out]
                        n2873 = Close File(refnum=w5311, error in=w5310) -> (error out=w5309:errorcluster)  [unwired: 1 out]
                        n2874 = local write "data file error"(w5309) -> ()
                      }
                      frame #1 {
                        n2875 = local read "JIG RELAY CYCLES"() -> (w5341:T8)
                        n2876 = Unbundle By Name(w5341) -> ("LAB01-1"=w5336:dbl, "LAB01-2"=w5335:dbl, "LAB02-1"=w5333:dbl, "LAB02-2"=w5332:dbl, "LAB03-1"=w5330:dbl, "LAB03-2"=w5327:dbl, "LAB04-1"=w5326:dbl, "LAB04-2"=w5324:dbl, "LAB05-1"=w5322:dbl, "LAB05-2"=w5320:dbl)
                        n2877 = stacked-sequence {
                          tunnel: w5336 -> [w5344 _ _ _ _ _ _ _ _ _]
                          tunnel: 1000000 -> [w5347 w5357 w5367 w5377 w5387 w5397 w5407 w5417 w5427 w5437]
                          tunnel: [w5345 _ _ _ _ _ _ _ _ _] -> w5339
                          tunnel: "TEST STATION HAS REACHED 1 MILLION CYCLES, REPLACE  CONTROL RELAYS" -> [w5343 w5355 w5365 w5375 w5385 w5395 w5405 w5415 w5425 w5435]
                          tunnel: [_ w5354 _ _ _ _ _ _ _ _] -> w5337
                          tunnel: w5335 -> [_ w5353 _ _ _ _ _ _ _ _]
                          tunnel: [_ _ w5364 _ _ _ _ _ _ _] -> w5334
                          tunnel: w5333 -> [_ _ w5363 _ _ _ _ _ _ _]
                          tunnel: w5332 -> [_ _ _ w5374 _ _ _ _ _ _]
                          tunnel: [_ _ _ w5373 _ _ _ _ _ _] -> w5331
                          tunnel: w5330 -> [_ _ _ _ w5384 _ _ _ _ _]
                          tunnel: [_ _ _ _ w5383 _ _ _ _ _] -> w5329
                          tunnel: [_ _ _ _ _ w5394 _ _ _ _] -> w5328
                          tunnel: w5327 -> [_ _ _ _ _ w5393 _ _ _ _]
                          tunnel: w5326 -> [_ _ _ _ _ _ w5404 _ _ _]
                          tunnel: [_ _ _ _ _ _ w5403 _ _ _] -> w5325
                          tunnel: w5324 -> [_ _ _ _ _ _ _ w5414 _ _]
                          tunnel: [_ _ _ _ _ _ _ w5413 _ _] -> w5323
                          tunnel: w5322 -> [_ _ _ _ _ _ _ _ w5424 _]
                          tunnel: [_ _ _ _ _ _ _ _ w5423 _] -> w5321
                          tunnel: w5320 -> [_ _ _ _ _ _ _ _ _ w5434]
                          tunnel: [_ _ _ _ _ _ _ _ _ w5433] -> w5319
                          frame #0 {
                            n2878 = Greater?(x=w5344, y=w5347) -> (0:w5346:bool)
                            n2879 = case shown="True" w5346 {
                              tunnel: [w5348 0] -> w5345
                              tunnel: w5344 -> [w5348 _]
                              tunnel: w5343 -> [_ w5349]
                              frame False {
                              }
                              frame True {
                                n2880 = Concatenate Strings("LA01-1 ", w5349) -> (w5352:string)
                                n2881 = One Button Dialog(message=w5352) -> ()  [unwired: 1 in, 1 out]
                              }
                            }
                          }
                          frame #1 {
                            n2882 = Greater?(x=w5353, y=w5357) -> (0:w5356:bool)
                            n2883 = case shown="True" w5356 {
                              tunnel: [w5358 0] -> w5354
                              tunnel: w5353 -> [w5358 _]
                              tunnel: w5355 -> [_ w5359]
                              frame False {
                              }
                              frame True {
                                n2884 = Concatenate Strings("LA01-2 ", w5359) -> (w5362:string)
                                n2885 = One Button Dialog(message=w5362) -> ()  [unwired: 1 in, 1 out]
                              }
                            }
                          }
                          frame #2 {
                            n2886 = Greater?(x=w5363, y=w5367) -> (0:w5366:bool)
